vi "Get VI Item in String.vi"(7 "items":T2(array[cluster]), 9 "Coords":T1, 11 "String in":refnum<vi>) -> (0 "item index":i32, 1 "active item":bool, 2 "item at coords":T3, 3 "String out":refnum<vi>)   [LabVIEW 2020, in "Explain Error Improved Dialog.lvlib"]
uses:
  Explain Error Improved Dialog/Explain Error Improved Dialog.lvlib
  <vilib>/Utility/miscctls.llb/LVPoint32TypeDef.ctl
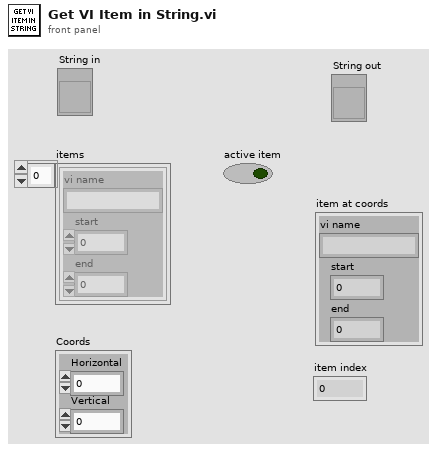
[diagram p1: front panel]
types:
  T1 = typedef "LVPoint32TypeDef.ctl" = cluster{"Horizontal":i32, "Vertical":i32}
  T2 = cluster{"vi name":string, "start":i32, "end":i32}[]
  T3 = cluster{"vi name":string, "start":i32, "end":i32}
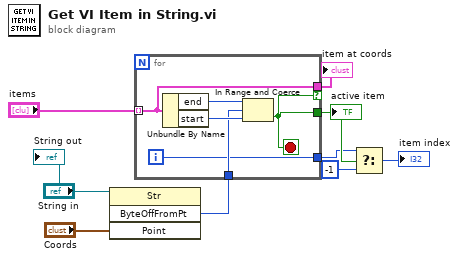
[diagram p0: block diagram]
diagram:
  n1 = invoke class="Str" method="ByteOffFromPt"(reference="String in", "Point"="Coords") -> ("ByteOffFromPt"=w8:i32)  [unwired: 2 in, 3 out]
  n2 = for {
    tunnel: "items" -> [w12] mode=indexing
    tunnel: w8 -> [w13]
    tunnel: [w12] -> w9 if=w11
    tunnel: [w11] -> w4
    tunnel: [w10] -> w3
    i -> [w10]
    stop <- w11 stop-if-true
    n3 = Unbundle By Name(w12) -> ("end"=w15:i32, "start"=w14:i32)
    n4 = In Range and Coerce(upper limit=w15, x=w13, lower limit=w14) -> (In Range?=w11:bool)  [unwired: 1 out]
  }
  "item at coords" <- w9
  "active item" <- w4
  n5 = Select(t=w3, s=w4, f=-1) -> (s? t:f=→"item index":i32)
  "String out" <- "String in"
